vi "Set Routing Channel State Configurations.vi"(8 "error in":errorcluster, 10 "state configurations":T1, 11 "routing channel in":T4 format="%.0x") -> (0 "error out":errorcluster, 3 "routing channel out":T4=18446744073709551615 format="%.0x")   [LabVIEW 2017, in "Routing and Faulting Scripting.lvlib"]
doc: "Removes and replaces all existing states in a routing channel with the input."
uses:
  Routing and Faulting Scripting.lvlib
  <vilib>/NI Veristand/Custom Device API/Custom Device Item Ref.ctl
  Shared/Channel States.ctl
  Shared/Routing State.ctl
  Shared/Connection.ctl
  NationalInstruments.VeriStand.SystemDefinitionAPI
  Constants/Scripting Constants.vi
  Utility/Connection to String.vi
  <vilib>/NI Veristand/Custom Device API/Custom Device API.lvlib
  Shared/Routing and Faulting Shared.lvlib
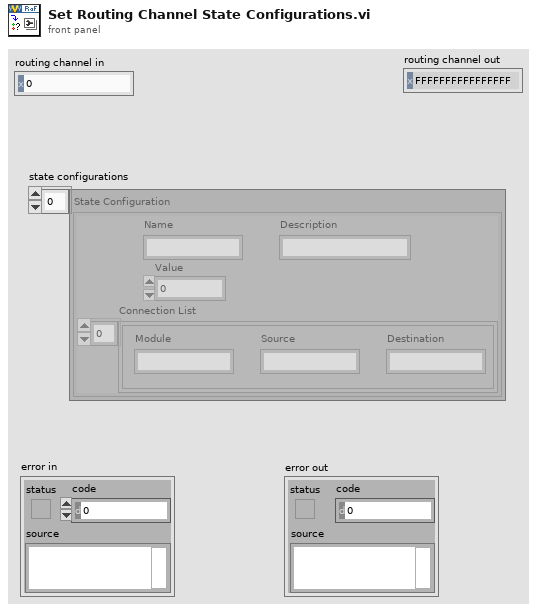
[diagram p1: front panel]
types:
  T1 = typedef "Routing and Faulting Shared.lvlib/Channel States.ctl" = T2[]
  T2 = typedef "Routing and Faulting Shared.lvlib/Routing State.ctl" = cluster{"Name":string, "Description":string, "Value":i32, "Connection List":T3[]}
  T3 = typedef "Routing and Faulting Shared.lvlib/Connection.ctl" = cluster{"Module":string, "Source":string, "Destination":string}
  T4 = typedef "Custom Device API.lvlib/Custom Device Item Ref.ctl" = u64
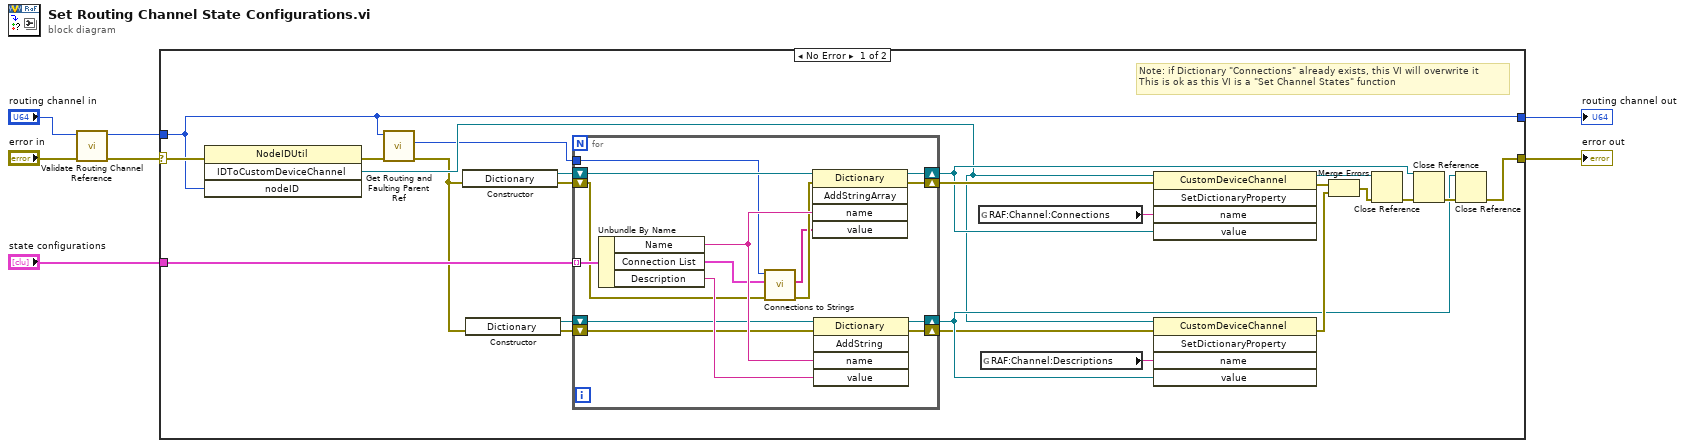
[diagram p0: block diagram]
diagram:
  n1 = call "Validate Routing Channel Reference.vi"("error in"="error in", "routing channel in"="routing channel in") -> ("error out"=w3:errorcluster, "routing channel out"=w1:T4)  [unwired: 8 in]
  n2 = case shown="No Error" w3 {
    selector: w3 -> [w31 w48]
    tunnel: [w30 w48] -> w6
    tunnel: w1 -> [w9 w47]
    tunnel: [w9 w47] -> w5
    tunnel: "state configurations" -> [w27 _]
    frame No Error {
      # "Note: if Dictionary \"Connections\" already exists, this VI will overwrite it\nThis is ok as this VI is a \"Set Channel States\" function"
      n3 = invoke class="NodeIDUtil" method="IDToCustomDeviceChannel"(error in=w31, "nodeID"=w9) -> (error out=w11:errorcluster, "IDToCustomDeviceChannel"=w12:refnum<k24>)  [unwired: 2 in, 2 out]
      n4 = call "Get Routing and Faulting Parent Ref.vi"("error in"=w11, "routing and faulting child in"=w9) -> ("error out"=w10:errorcluster, "routing and faulting"=w8:T4)  [unwired: 7 in, 1 out]
      n5 = constructor class="Dictionary"(error in=w10) -> (reference out=w26:refnum<k24>, error out=w14:errorcluster)  [unwired: 2 in, 1 out]
      n6 = constructor class="Dictionary"(error in=w10) -> (reference out=w25:refnum<k24>, error out=w15:errorcluster)  [unwired: 2 in, 1 out]
      n7 = for {
        tunnel: w27 -> [w46] mode=indexing
        shift-right: [w39] -> w22
        shift-left: w14 -> [w35]
        shift-right: [w43] -> w17
        shift-left: w25 -> [w41]
        shift-right: [w42] -> w18
        shift-left: w26 -> [w40]
        shift-right: [w38] -> w13
        shift-left: w15 -> [w36]
        tunnel: w8 -> [w32]
        n8 = Unbundle By Name(w46) -> ("Name"=w45:string, "Connection List"=w37:T3[], "Description"=w44:string)
        n9 = call "Connections to Strings.vi"("error in"=w35, "connection list"=w37, "routing and faulting in"=w32) -> ("error out"=w34:errorcluster, "connection strings"=w33:string[])  [unwired: 6 in, 1 out]
        n10 = invoke class="Dictionary" method="AddStringArray"(reference=w40, error in=w34, "name"=w45, "value"=w33) -> (reference out=w42:refnum<k24>, error out=w39:errorcluster)  [unwired: 1 in, 3 out]
        n11 = invoke class="Dictionary" method="AddString"(reference=w41, error in=w36, "name"=w45, "value"=w44) -> (reference out=w43:refnum<k24>, error out=w38:errorcluster)  [unwired: 1 in, 3 out]
      }
      n12 = global read "Scripting Constants.vi" "RAF:Channel:Connections"() -> (w28:string)
      n13 = global read "Scripting Constants.vi" "RAF:Channel:Descriptions"() -> (w16:string)
      n14 = invoke class="CustomDeviceChannel" method="SetDictionaryProperty"(reference=w12, error in=w22, "name"=w28, "value"=w18) -> (reference out=w29:refnum<k24>, error out=w20:errorcluster)  [unwired: 1 in, 3 out]
      n15 = invoke class="CustomDeviceChannel" method="SetDictionaryProperty"(reference=w12, error in=w13, "name"=w16, "value"=w17) -> (error out=w21:errorcluster)  [unwired: 1 in, 4 out]
      n16 = Merge Errors(w20, w21) -> (w19:errorcluster)
      n17 = Close Reference(reference=w29, error in (no error)=w19) -> (error out=w24:errorcluster)
      n18 = Close Reference(reference=w18, error in (no error)=w24) -> (error out=w23:errorcluster)
      n19 = Close Reference(reference=w17, error in (no error)=w23) -> (error out=w30:errorcluster)
    }
    frame Error {
    }
  }
  "routing channel out" <- w5
  "error out" <- w6
